vi "Settings_Config.vi"(11 "DataCluster in":T1={"Core"={"Current VI Reference"=refnum, "Close Panel on Exit?"=FALSE, "Exit"=FALSE}, "Connections"={"cDAQ Therm"={"Task"="", "Connected"=FALSE, "Active"=FALSE}, "cDAQ Voltage"={"Task"="", "Connected"=FALSE, "Active"=FALSE}, "Camera"={"Session"="", "Connected"=FALSE, "Active"=FALSE}}, "Data Acquisition"={"Setup"={"Label"="", "Operator"="", "Notes"="", "TempGrad"=1.0, "TargetTemp"=1.0, "Sample Volume"=1.0}, "Camera"={"Image"=refnum, "Save Image"=refnum}, "Thermistor"={"Sample Size"=1, "Calibration"={"B0.100"=[], "R25"=[], "V_S"=5.0, "R_S"=100.0}, "Timing Mode"=14713}, "Queue"={"Size"=1, "Queue"=refnum}, "Sample Rate"=1, "Active"=FALSE, "Ready"=FALSE, "Partition"={"Data"=[], "Cell Label"="", "Cell Color"=0, "Height"=10, "Width"=16, "Grid"=[]}}, "Control"={"Sample Rate"=1, "PID gains"={"proportional gain (Kc)"=1.0, "integral time (Ti, min)"=0.01, "derivative time (Td, min)"=0.0}}} {"Control"."PID gains"."derivative time (Td, min)" format="%.3f"; "Control"."PID gains"."integral time (Ti, min)" format="%.3f"; "Control"."PID gains"."proportional gain (Kc)" format="%.3f"; "Control"."Sample Rate" min=1 max=20 step=1 format="%.0f Samples/sec"; "Data Acquisition"."Thermistor"."Timing Mode" items=["Automatic"=16097, "High Resolution"=10195, "High Speed"=14712, "Best 50 Hz Rejection"=14713, "Best 60 Hz Rejection"=14714, "Custom"=10137]; "Data Acquisition"."Thermistor"."Calibration"."R_S" min=0.1 max=1000.0 format="%#_g kOhm"; "Data Acquisition"."Thermistor"."Calibration"."V_S" min=5.0 max=48.0 format="%#_g V"; "Data Acquisition"."Thermistor"."Calibration"."R25" min=0.1 max=1000.0 format="%#_g kOhm"; "Data Acquisition"."Thermistor"."Calibration"."B0.100" min=100.0 max=10000.0 format="%#_g K"; "Data Acquisition"."Thermistor"."Sample Size" min=1 max=200; "Data Acquisition"."Sample Rate" min=20 max=240 format="%.0f samples/min"; "Data Acquisition"."Queue"."Size" min=1 max=200; "Data Acquisition"."Setup"."Sample Volume" min=0.0 max=500.0 format="%#_g µL"; "Data Acquisition"."Setup"."TargetTemp" min=-30.0 max=30.0 step=0.5 format="%#_g °C"; "Data Acquisition"."Setup"."TempGrad" min=-100.0 max=100.0 step=0.1 format="%#_g °C/min"}) -> (3 "DataCluster out":T1={"Core"={"Current VI Reference"=refnum, "Close Panel on Exit?"=FALSE, "Exit"=FALSE}, "Connections"={"cDAQ Therm"={"Task"="", "Connected"=FALSE, "Active"=FALSE}, "cDAQ Voltage"={"Task"="", "Connected"=FALSE, "Active"=FALSE}, "Camera"={"Session"="", "Connected"=FALSE, "Active"=FALSE}}, "Data Acquisition"={"Setup"={"Label"="", "Operator"="", "Notes"="", "TempGrad"=1.0, "TargetTemp"=1.0, "Sample Volume"=1.0}, "Camera"={"Image"=refnum, "Save Image"=refnum}, "Thermistor"={"Sample Size"=1, "Calibration"={"B0.100"=[], "R25"=[], "V_S"=5.0, "R_S"=100.0}, "Timing Mode"=14713}, "Queue"={"Size"=1, "Queue"=refnum}, "Sample Rate"=1, "Active"=FALSE, "Ready"=FALSE, "Partition"={"Data"=[], "Cell Label"="", "Cell Color"=0, "Height"=10, "Width"=16, "Grid"=[]}}, "Control"={"Sample Rate"=1, "PID gains"={"proportional gain (Kc)"=1.0, "integral time (Ti, min)"=0.01, "derivative time (Td, min)"=0.0}}} {"Control"."PID gains"."derivative time (Td, min)" format="%.3f"; "Control"."PID gains"."integral time (Ti, min)" format="%.3f"; "Control"."PID gains"."proportional gain (Kc)" format="%.3f"; "Control"."Sample Rate" min=1 max=20 step=1 format="%.0f Samples/sec"; "Data Acquisition"."Thermistor"."Timing Mode" items=["Automatic"=16097, "High Resolution"=10195, "High Speed"=14712, "Best 50 Hz Rejection"=14713, "Best 60 Hz Rejection"=14714, "Custom"=10137]; "Data Acquisition"."Thermistor"."Calibration"."R_S" min=0.1 max=1000.0 format="%#_g kOhm"; "Data Acquisition"."Thermistor"."Calibration"."V_S" min=5.0 max=48.0 format="%#_g V"; "Data Acquisition"."Thermistor"."Calibration"."R25" min=0.1 max=1000.0 format="%#_g kOhm"; "Data Acquisition"."Thermistor"."Calibration"."B0.100" min=100.0 max=10000.0 format="%#_g K"; "Data Acquisition"."Thermistor"."Sample Size" min=1 max=200; "Data Acquisition"."Sample Rate" min=20 max=240 format="%.0f samples/min"; "Data Acquisition"."Queue"."Size" min=1 max=200; "Data Acquisition"."Setup"."Sample Volume" min=0.0 max=500.0 format="%#_g µL"; "Data Acquisition"."Setup"."TargetTemp" min=-30.0 max=30.0 step=0.5 format="%#_g °C"; "Data Acquisition"."Setup"."TempGrad" min=-100.0 max=100.0 step=0.1 format="%#_g °C/min"})   [LabVIEW 2020]
uses:
  DataCluster.ctl
  <vilib>/userDefined/High Color/IMAQdx.ctl
  <vilib>/vision/Image Controls.llb/IMAQ Image.ctl
panel:
  in  "Sample Volume":dbl=1.0 min=0.0 max=500.0 format="%#_g µL"
  in  "Sample Rate":i32=20 min=20 max=240 step=1 format="%.0f Samples/min"
  in  "Target Temperature":dbl=1.0 min=-30.0 max=30.0 step=0.5 format="%#_g °C"
  in  "OK":bool
  in  "Cancel":bool
  in  "Temperature Gradient":dbl=1.0 min=-100.0 max=100.0 step=0.1 format="%#_g °C/min"
  in  "Notes":string
  in  "Operator":string
  in  "Label":string
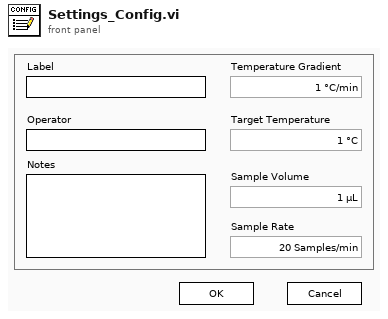
[diagram p1: front panel]
types:
  T1 = typedef "DataCluster.ctl" = cluster{"Core":cluster{"Current VI Reference":refnum<vi>, "Close Panel on Exit?":bool, "Exit":bool}, "Connections":cluster{"cDAQ Therm":cluster{"Task":refnum<k21>, "Connected":bool, "Active":bool}, "cDAQ Voltage":cluster{"Task":refnum<k21>, "Connected":bool, "Active":bool}, "Camera":cluster{"Session":T2, "Connected":bool, "Active":bool}}, "Data Acquisition":cluster{"Setup":cluster{"Label":string, "Operator":string, "Notes":string, "TempGrad":dbl, "TargetTemp":dbl, "Sample Volume":dbl}, "Camera":cluster{"Image":T3, "Save Image":T3}, "Thermistor":cluster{"Sample Size":i32, "Calibration":cluster{"B0.100":dbl[], "R25":dbl[], "V_S":dbl, "R_S":dbl}, "Timing Mode":i32}, "Queue":cluster{"Size":i32, "Queue":refnum<queue>}, "Sample Rate":i32, "Active":bool, "Ready":bool, "Partition":cluster{"Data":string[][], "Cell Label":string, "Cell Color":u32, "Height":i32, "Width":i32, "Grid":string[][]}}, "Control":cluster{"Sample Rate":i32, "PID gains":cluster{"proportional gain (Kc)":dbl, "integral time (Ti, min)":dbl, "derivative time (Td, min)":dbl}}}
  T2 = typedef "IMAQdx.ctl" = refnum<k21>
  T3 = typedef "IMAQ Image.ctl" = refnum<image>
  T4 = enum8{"Enabled", "Disabled", "Disabled and Grayed Out"}
  T5 = cluster{"Label":string, "Operator":string, "Notes":string, "TempGrad":dbl, "TargetTemp":dbl, "Sample Volume":dbl}
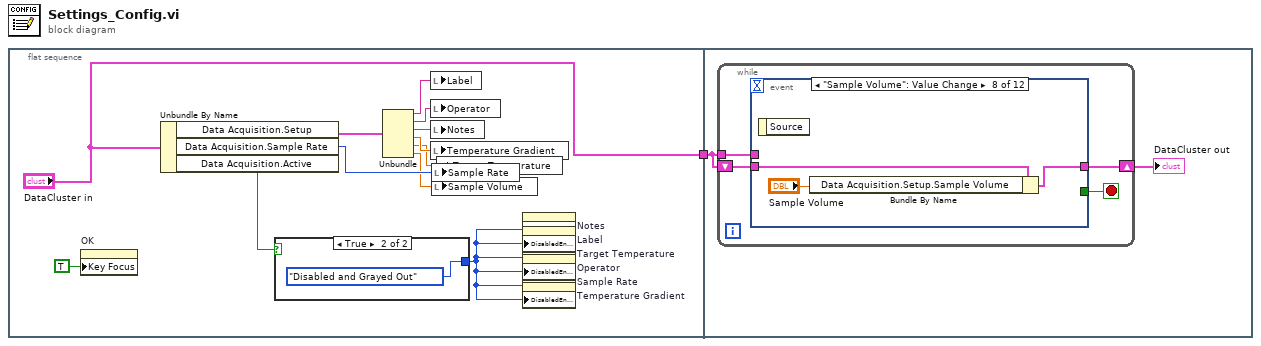
[diagram p0: block diagram]
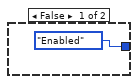
[diagram p2: hidden frame]
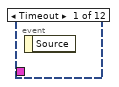
[diagram p3: hidden frame]
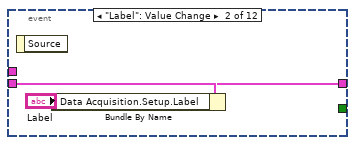
[diagram p4: hidden frame]
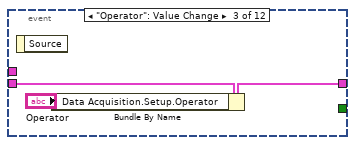
[diagram p5: hidden frame]
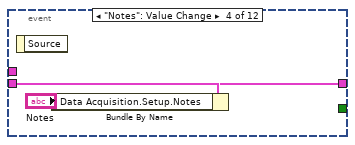
[diagram p6: hidden frame]
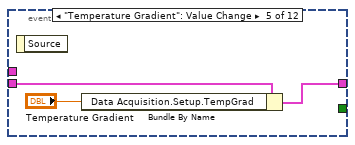
[diagram p7: hidden frame]
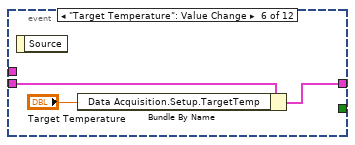
[diagram p8: hidden frame]
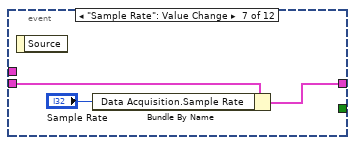
[diagram p9: hidden frame]
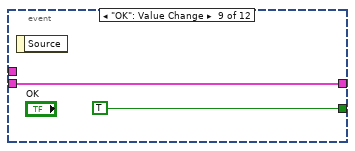
[diagram p10: hidden frame]
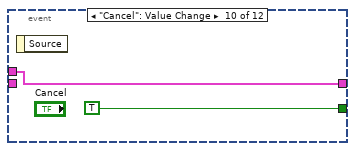
[diagram p11: hidden frame]
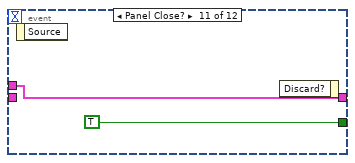
[diagram p12: hidden frame]
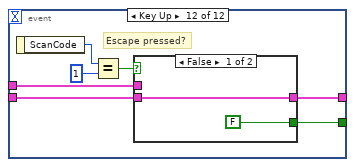
[diagram p13: hidden frame]
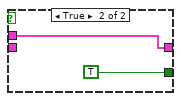
[diagram p14: hidden frame]
diagram:
  n1 = flat-sequence {
    tunnel: ["DataCluster in"] -> w1
    tunnel: w1 -> [w17]
    frame #0 {
      n2 = property on="OK" class="Bool"("Key Focus"=TRUE) -> ()  [unwired: 2 in, 2 out]
      n3 = Unbundle By Name("DataCluster in") -> ("Data Acquisition.Setup"=w13:T5, "Data Acquisition.Sample Rate"=w5:i32, "Data Acquisition.Active"=w6:bool)
      n4 = case shown="True" w6 {
        tunnel: [T4."Enabled" ("Disabled") T4."Disabled and Grayed Out" ("Disabled")] -> w2
        frame False {
        }
        frame True {
        }
      }
      n5 = Unbundle(w13) -> ("Label"=w12:string, "Operator"=w8:string, "Notes"=w7:string, "TempGrad"=w11:dbl, "TargetTemp"=w3:dbl, "Sample Volume"=w4:dbl)
      n6 = local write "Label"(w12) -> ()
      n7 = local write "Operator"(w8) -> ()
      n8 = local write "Notes"(w7) -> ()
      n9 = local write "Temperature Gradient"(w11) -> ()
      n10 = local write "Sample Rate"(w5) -> ()
      n11 = local write "Sample Volume"(w4) -> ()
      n12 = local write "Target Temperature"(w3) -> ()
      n13 = property on="Notes" class="Str"("DisabledEnum"=w2) -> ()  [unwired: 2 in, 2 out]
      n14 = property on="Label" class="Str"("DisabledEnum"=w2) -> ()  [unwired: 2 in, 2 out]
      n15 = property on="Target Temperature" class="DigNum (strict)"("DisabledEnum"=w2) -> ()  [unwired: 2 in, 2 out]
      n16 = property on="Operator" class="Str"("DisabledEnum"=w2) -> ()  [unwired: 2 in, 2 out]
      n17 = property on="Sample Rate" class="DigNum (strict)"("DisabledEnum"=w2) -> ()  [unwired: 2 in, 2 out]
      n18 = property on="Temperature Gradient" class="DigNum (strict)"("DisabledEnum"=w2) -> ()  [unwired: 2 in, 2 out]
    }
    frame #1 {
      n19 = while {
        shift-right: [w21] -> w16
        shift-left: w17 -> [w20]
        tunnel: w17 -> [w19]
        stop <- w18 stop-if-true
        n20 = event shown="[7] \"Sample Volume\": Value Change" {
          selector: _ -> [_ _ _ _ _ _ _ _ _ _ _ _]
          dyn-events: _ -> [_ _ _ _ _ _ _ _ _ _ _ _]
          timeout: _ -> [_ _ _ _ _ _ _ _ _ _ _ _]
          tunnel: w20 -> [_ w24 w27 w30 w33 w36 w39 w42 w44 _ _ w49]
          tunnel: [_ w23 w26 w29 w32 w35 w38 w41 w44 w46 w48 w51] -> w21
          tunnel: w19 -> [_ _ _ _ _ _ _ _ _ w46 w48 w50]
          tunnel: [_ _ _ _ _ _ _ _ TRUE TRUE TRUE w55] -> w18
          event Timeout {
            n21 = event-data() -> ()  [unwired: 1 in, 1 out]
          }
          event "Label": Value Change {
            n22 = event-data() -> ()  [unwired: 1 in, 1 out]
            n23 = Bundle By Name(cluster=w24, "Data Acquisition.Setup.Label"="Label") -> (w23:T1)
          }
          event "Operator": Value Change {
            n24 = event-data() -> ()  [unwired: 1 in, 1 out]
            n25 = Bundle By Name(cluster=w27, "Data Acquisition.Setup.Operator"="Operator") -> (w26:T1)
          }
          event "Notes": Value Change {
            n26 = event-data() -> ()  [unwired: 1 in, 1 out]
            n27 = Bundle By Name(cluster=w30, "Data Acquisition.Setup.Notes"="Notes") -> (w29:T1)
          }
          event "Temperature Gradient": Value Change {
            n28 = event-data() -> ()  [unwired: 1 in, 1 out]
            n29 = Bundle By Name(cluster=w33, "Data Acquisition.Setup.TempGrad"="Temperature Gradient") -> (w32:T1)
          }
          event "Target Temperature": Value Change {
            n30 = event-data() -> ()  [unwired: 1 in, 1 out]
            n31 = Bundle By Name(cluster=w36, "Data Acquisition.Setup.TargetTemp"="Target Temperature") -> (w35:T1)
          }
          event "Sample Rate": Value Change {
            n32 = event-data() -> ()  [unwired: 1 in, 1 out]
            n33 = Bundle By Name(cluster=w39, "Data Acquisition.Sample Rate"="Sample Rate") -> (w38:T1)
          }
          event "Sample Volume": Value Change {
            n34 = event-data() -> ()  [unwired: 1 in, 1 out]
            n35 = Bundle By Name(cluster=w42, "Data Acquisition.Setup.Sample Volume"="Sample Volume") -> (w41:T1)
          }
          event "OK": Value Change {
            n36 = event-data() -> ()  [unwired: 1 in, 1 out]
          }
          event "Cancel": Value Change {
            n37 = event-data() -> ()  [unwired: 1 in, 1 out]
          }
          event Panel Close? {
            n38 = event-data() -> ()  [unwired: 1 in, 1 out]
            n39 = event-data() -> ()  [unwired: 2 in, 1 out]
          }
          event Key Up {
            # "Escape pressed?"
            n40 = event-data() -> ("ScanCode"=w54:i16)  [unwired: 1 in]
            n41 = Equal?(x=w54, y=i16 1) -> (x = y?=w52:bool)
            n42 = case shown="False" w52 {
              tunnel: [FALSE TRUE] -> w55
              tunnel: [w57 w58] -> w51
              tunnel: w50 -> [_ w58]
              tunnel: w49 -> [w57 _]
              frame False {
              }
              frame True {
              }
            }
          }
        }
      }
      "DataCluster out" <- w16
    }
  }
